vi "ReadConcTempPressureVer08.vi"() -> ()   [LabVIEW 2011]
uses:
  <vilib>/Utility/error.llb/DialogType.ctl
  <vilib>/Analysis/NI_AALBase.lvlib
panel:
  out "CavityTemperature":dbl
  out "CavityPressure":dbl
  in  "Measurment Type":T1(ring)=enum."Particles Measurement"
  out "CPCconc":dbl=nan
  out "Smps Setting String":string
  out "Saving in Progress":i32(slide) caption="Saving" scale=0.0..9.0
  out "P (Hectopascal)":dbl=1014.187137206139 format="%#.2f"
  out "Mean P":dbl=1014.4104948184322 format="%.1f"
  out "Std Error P (%)":dbl=0.009142669652284326 format="%.2f"
  out "Number Samples of Press.":dbl format="%.1f"
  out "Std error Press. to file (hpas)":dbl format="%.2f"
  out "Mean Press. to file (hpas)":dbl format="%.2f"
  in  "Std Press. error tolerance(%)":dbl=0.1 format="%.1f"
  out "Pressure Graph":waveform(dbl)[](graph)=[{"t0"=timestamp(3472445026.4531226 s since 1904-01-01), "dt"=1.0, "Y"=[1014.187137206139]}, {"t0"=timestamp(3472445026.4531226 s since 1904-01-01), "dt"=1.0, "Y"=[1014.4104948184322]}] caption="Waveform Chart"
  out "Temp (C)":dbl=23.130823558220463 format="%#.2f"
  out "Mean Temp":dbl=23.127451250466187 format="%.2f"
  out "Std Error T (%)":dbl=0.012599717898815081 format="%.2f"
  out "Number Samples of Temp":dbl format="%.1f"
  out "Std error Temp to file (deg)":dbl format="%.1f"
  out "Mean Temp to file (deg)":dbl format="%#.0f"
  in  "Std Temp error tolerance(%)":dbl=0.1 format="%.1f"
  out "Temperature Graph":waveform(dbl)[](graph)=[{"t0"=timestamp(3472445026.4531226 s since 1904-01-01), "dt"=1.0, "Y"=[23.130823558220463]}, {"t0"=timestamp(3472445026.4531226 s since 1904-01-01), "dt"=1.0, "Y"=[23.127451250466187]}] caption="Waveform Chart"
  in  "CPC port":refnum<visa-resource-name>="COM1"
  out "Conc. (N/cm^3)":dbl=nan format="%.1f"
  out "Mean Conc.":dbl=nan format="%.1f"
  out "Std Error Conc. (%)":dbl=nan format="%.2f"
  out "Number Samples of Conc.":dbl format="%.1f"
  out "Std error to file (N/cm^3)":dbl format="%.1f"
  out "Mean conc. to file (N/cm^3)":dbl format="%.2f"
  out "output array 2":dbl[](array[numeric])
  out "output 2":dbl
  out "output 1":dbl
  out "Std Error Concentration":dbl=nan format="%.1f"
  in  "Std Conc. error tolerance(%)":dbl=1.0 format="%.1f"
  out "Std Concentration":dbl=nan format="%.1f"
  out "output array":dbl[](array[numeric])=[nan, nan, nan, nan, nan, nan, nan, nan, nan, nan, nan, 0.0, 0.0, 0.0, 0.0, 1.0, 1.0, 1.0, 0.0, 0.0, 0.0, 0.0, 0.0, 0.0, 0.0, 0.0, 0.0, nan, nan, nan]
  in  "Running Average Time(sec)":i32=30
  out "Particle Concentration from CPC":waveform(dbl)[](graph)=[{"t0"=timestamp(3472445026.4531226 s since 1904-01-01), "dt"=1.0, "Y"=[nan]}, {"t0"=timestamp(3472445026.4531226 s since 1904-01-01), "dt"=1.0, "Y"=[nan]}] caption="Waveform Chart"
  in  "OK":bool
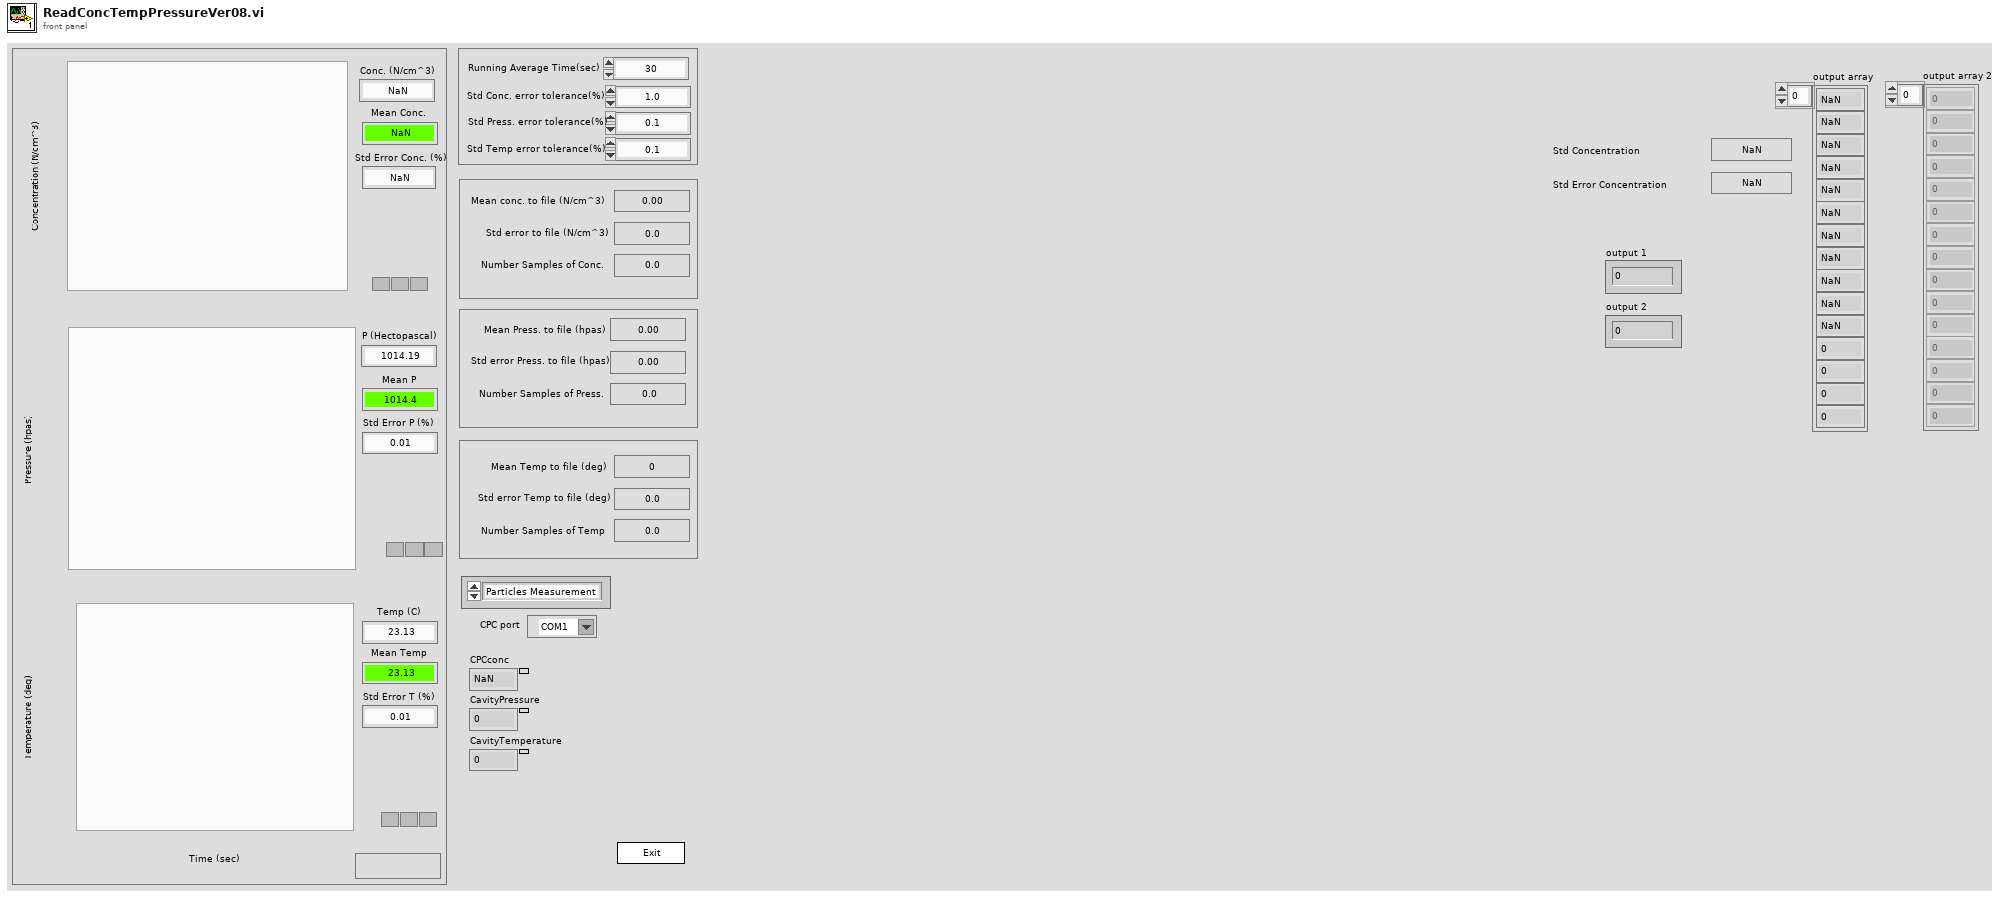
[diagram p1: front panel]
types:
  T1 = enum16{"Gas Measurement", "Particles Measurement", "SMPS scan"}
  T2 = enum32{"invalid app kind", "Development System", "Run Time System", "Student Edition", "Embedded LabVIEW", "Evaluation", "Custom"}
  T3 = enum32{"Invalid", "Standard", "Closed", "Hidden", "Minimized", "Maximized"}
  T4 = cluster{"Core":cluster{"Current VI Reference":refnum<vi>, "Close Panel on Exit?":bool}, dbl[], "Running Average Time(sec)":i32, dbl[], "element":dbl, "dimension size":i32, "input file":path, "input file":path, "dup CPC port":refnum<visa-resource-name>, "CPC model":string, "input file":path, "input file":path, cluster{dbl[], dbl[], "element":dbl}, cluster{dbl[], dbl[], "element":dbl}}
  T5 = typedef "DialogType.ctl" = u16
  T6 = cluster{"Current VI Reference":refnum<vi>, "Close Panel on Exit?":bool}
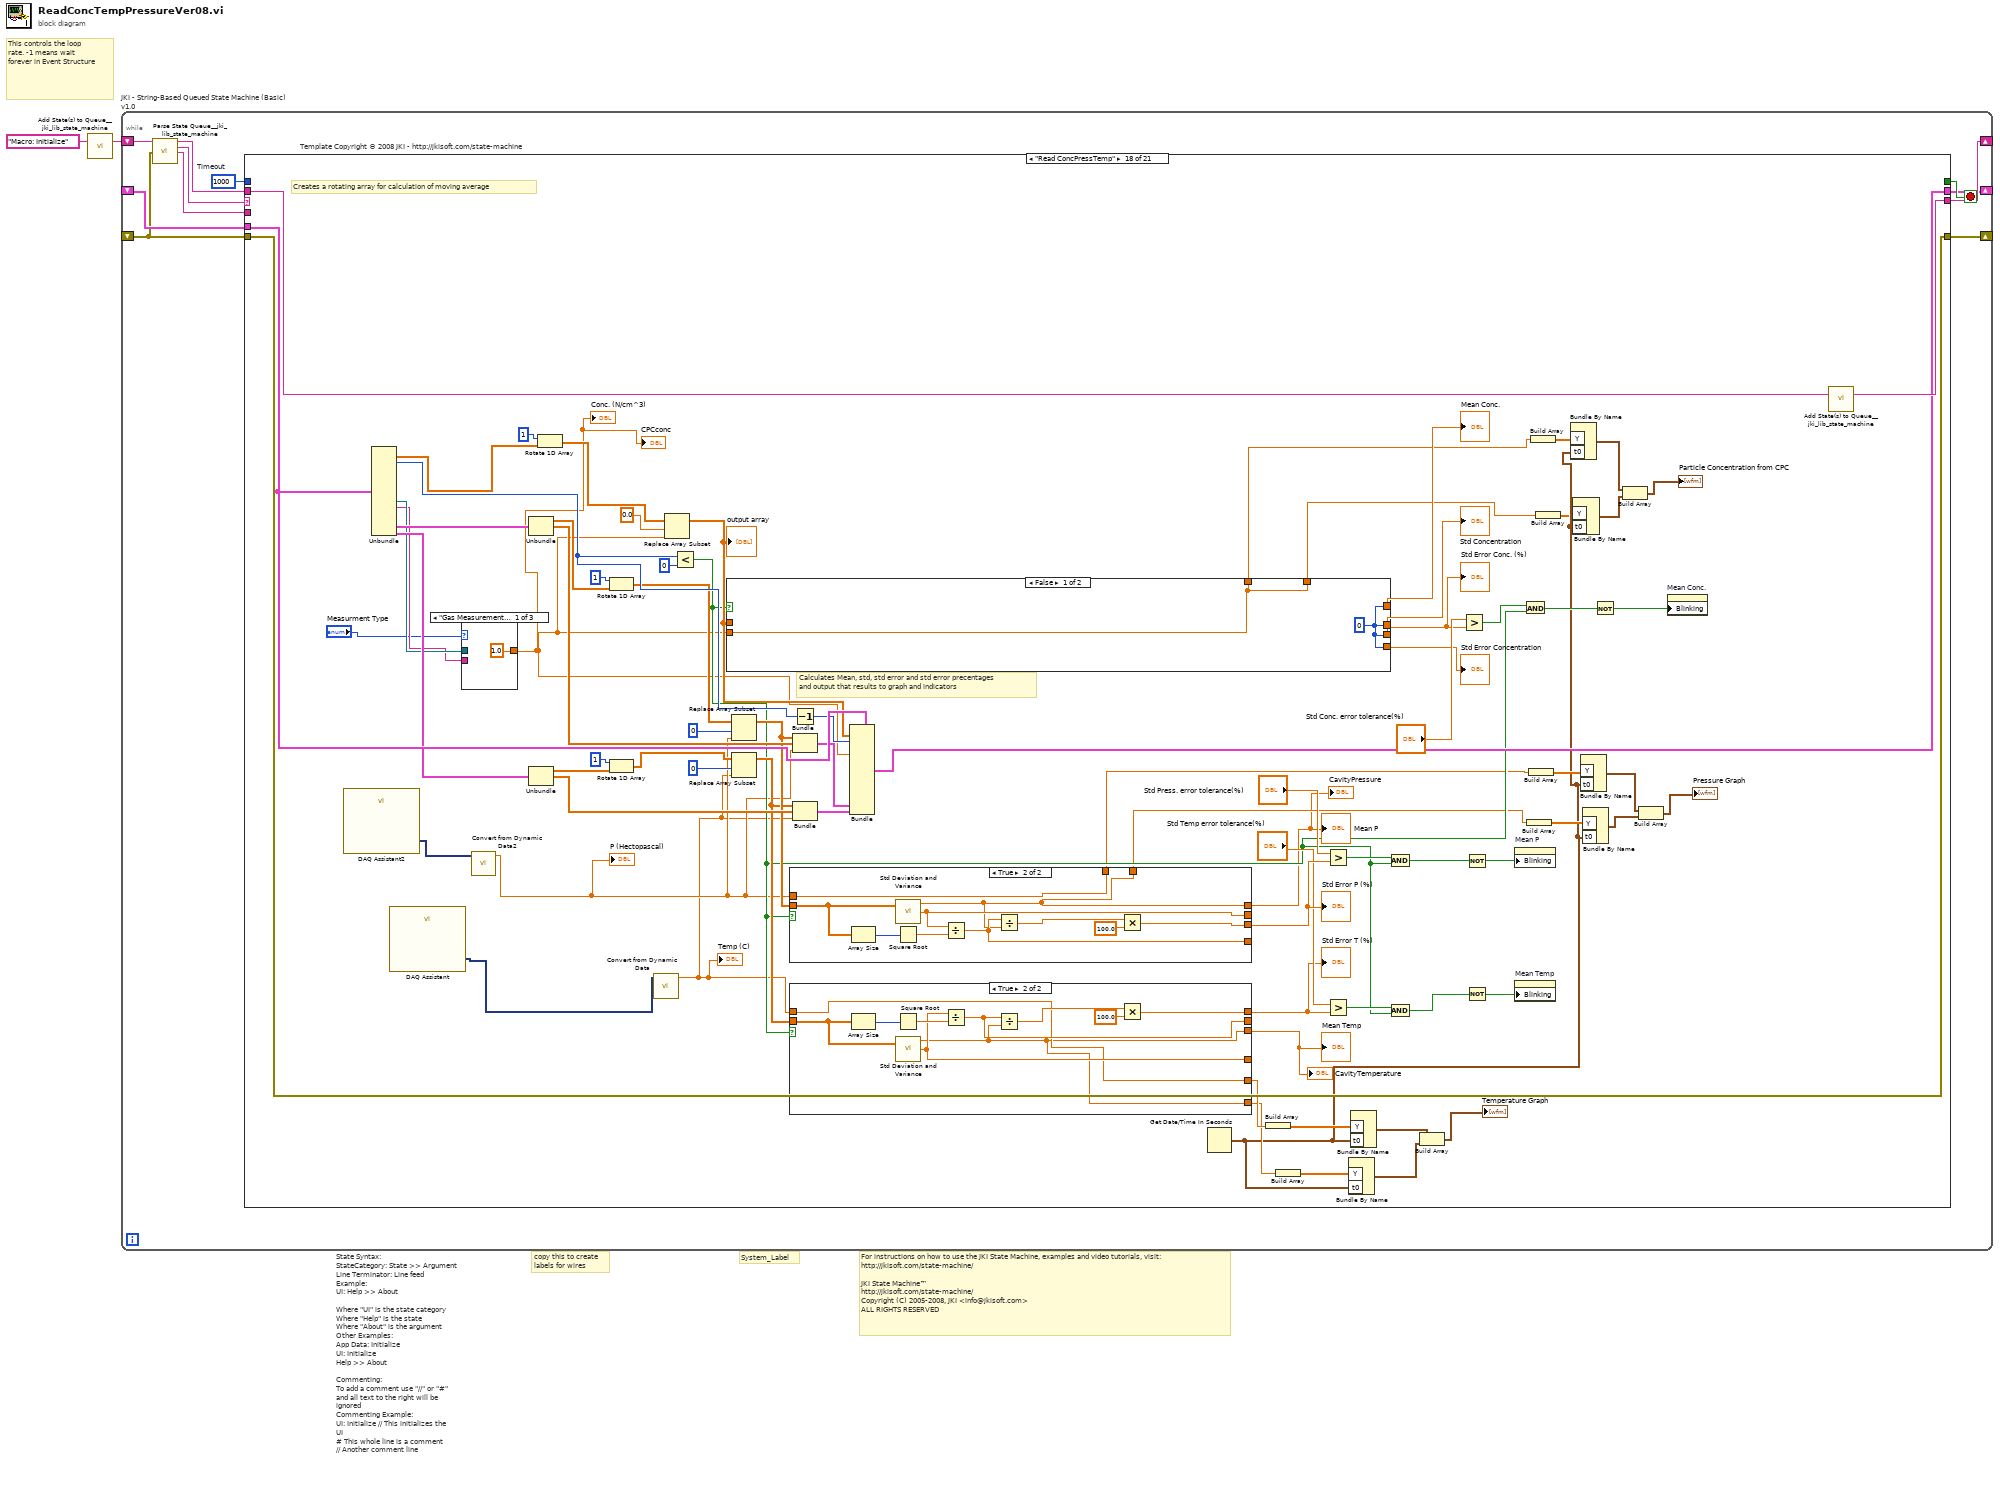
[diagram p0: block diagram]
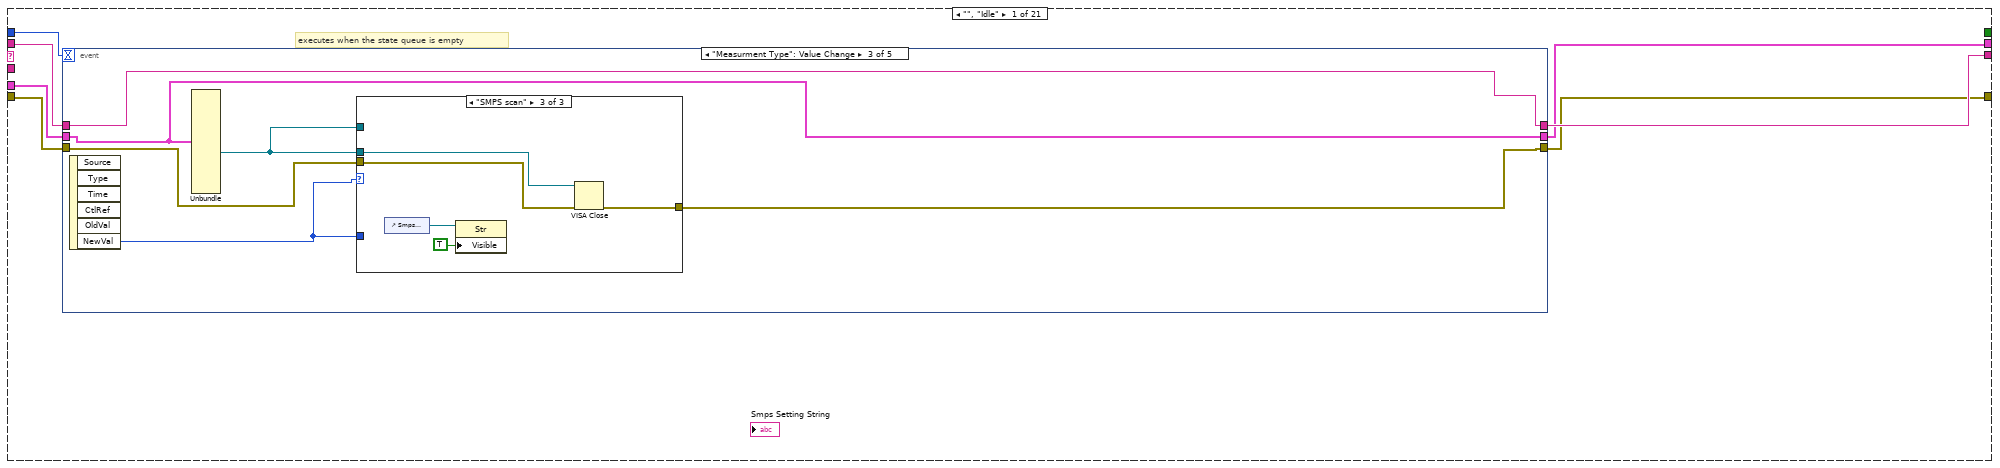
[diagram p2: hidden frame]
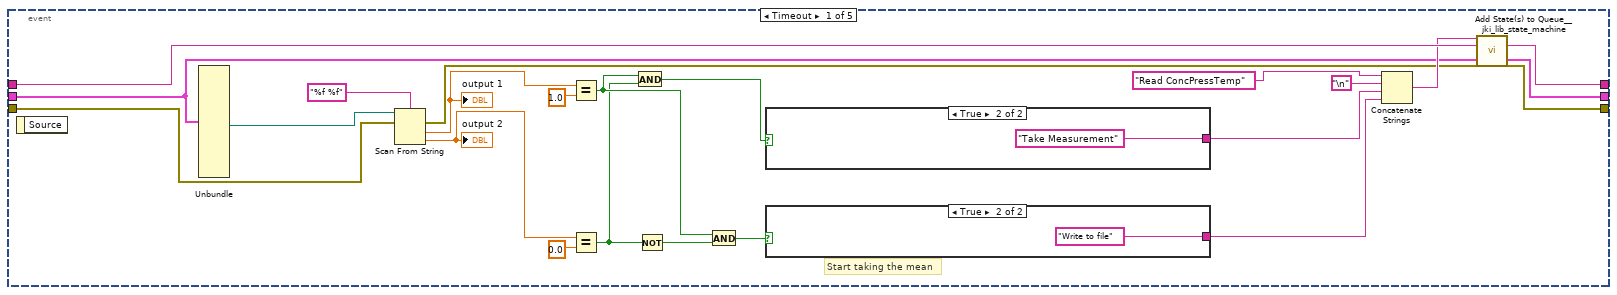
[diagram p3: hidden frame]
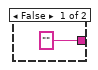
[diagram p4: hidden frame]
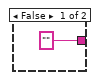
[diagram p5: hidden frame]
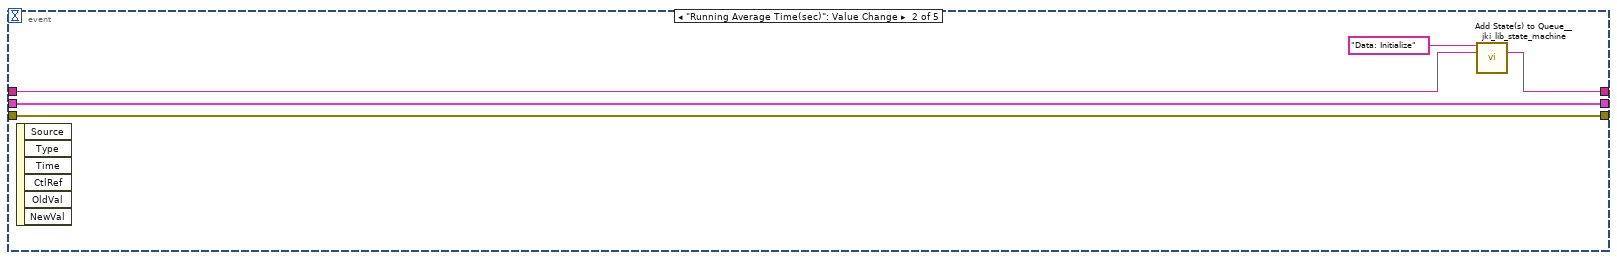
[diagram p6: hidden frame]
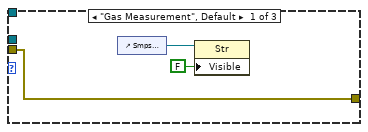
[diagram p7: hidden frame]
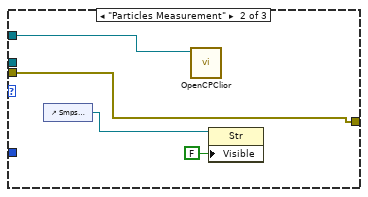
[diagram p8: hidden frame]
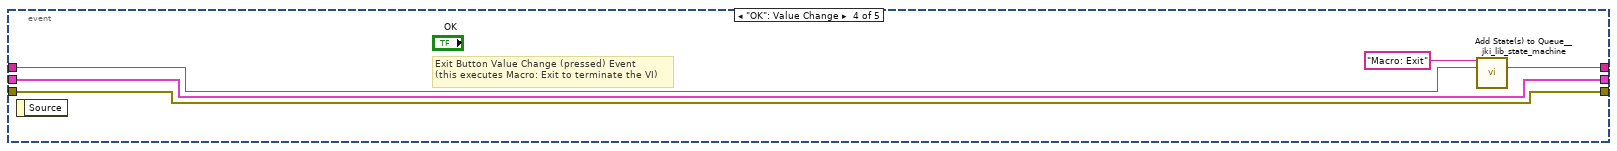
[diagram p9: hidden frame]
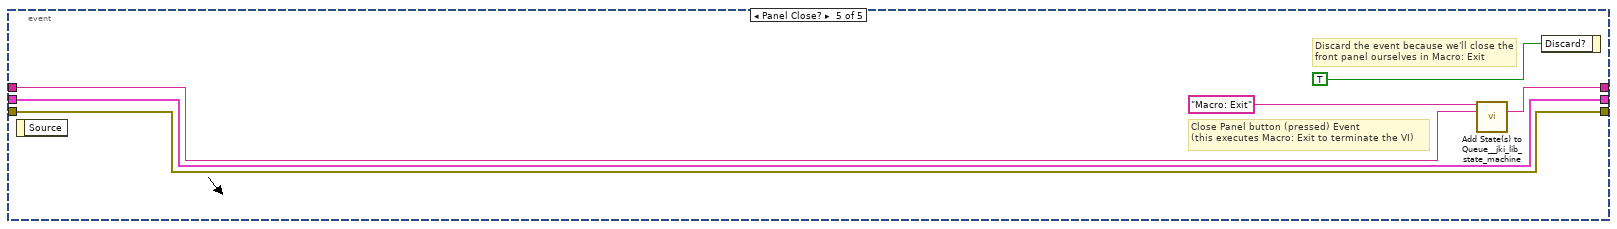
[diagram p10: hidden frame]
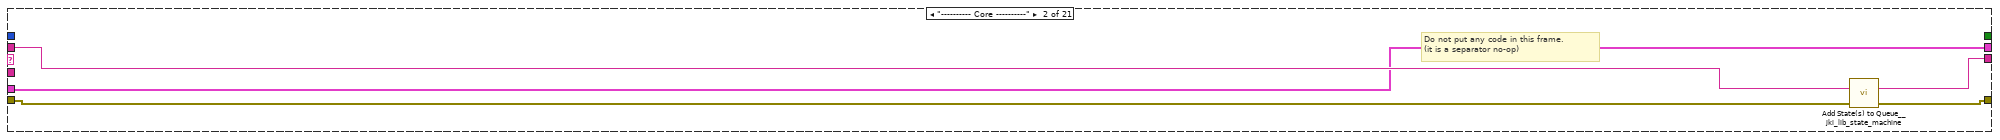
[diagram p11: hidden frame]
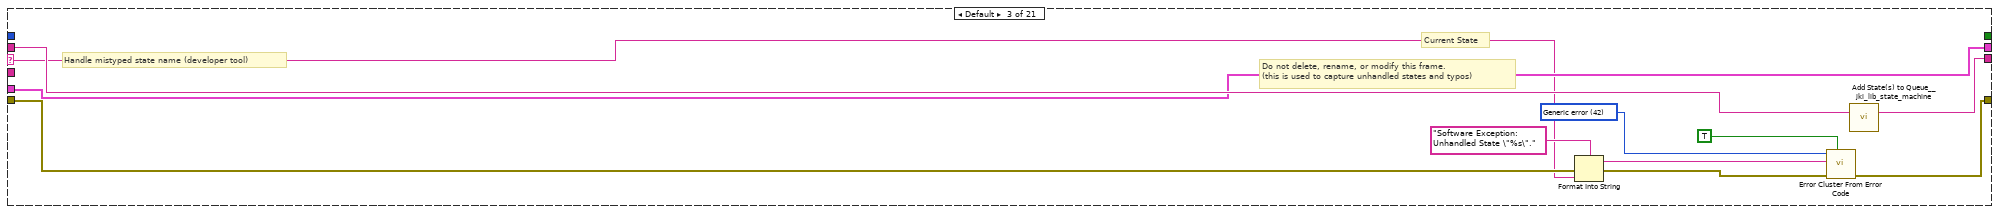
[diagram p12: hidden frame]
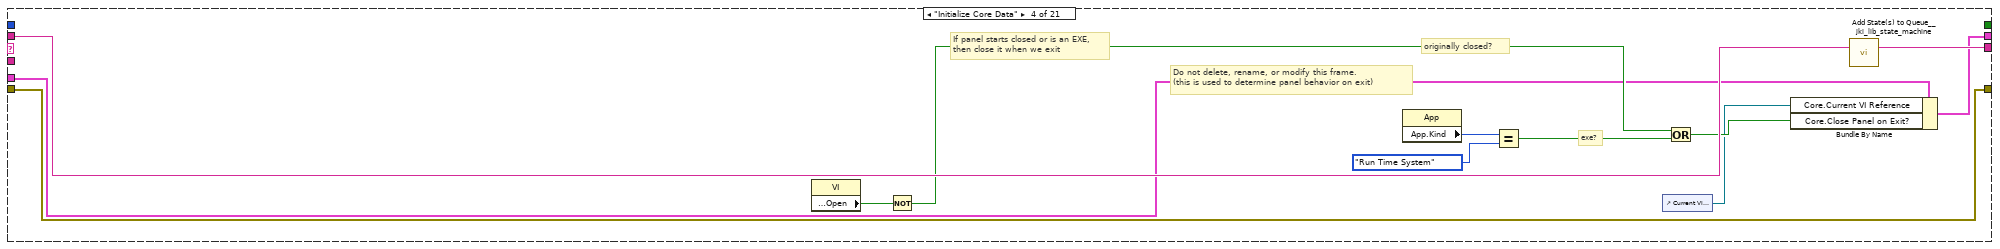
[diagram p13: hidden frame]
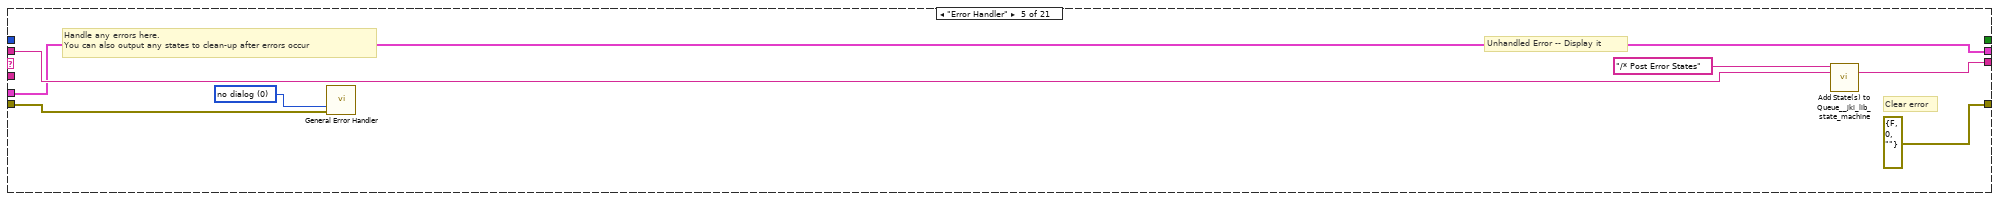
[diagram p14: hidden frame]
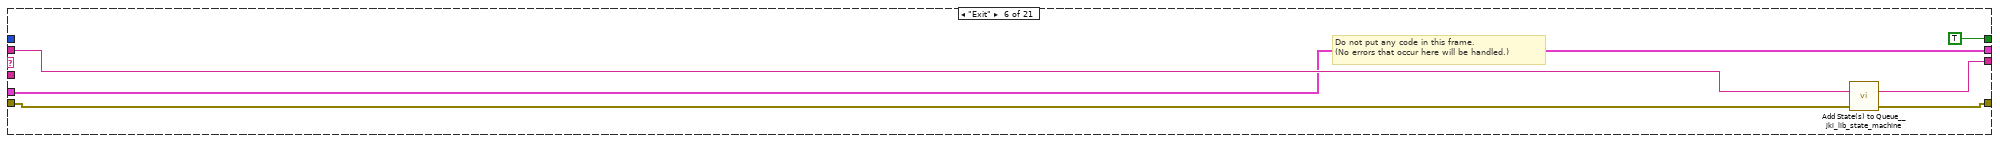
[diagram p15: hidden frame]
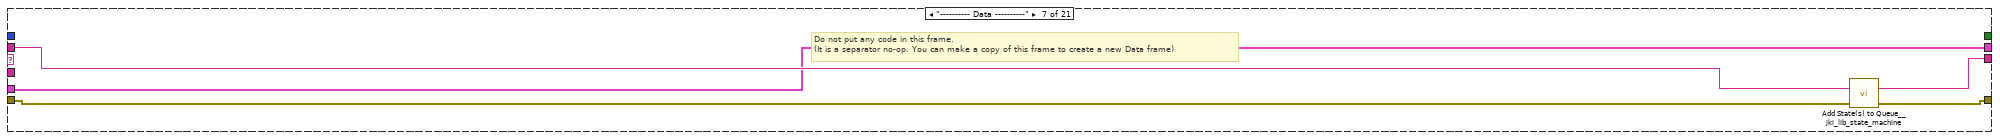
[diagram p16: hidden frame]
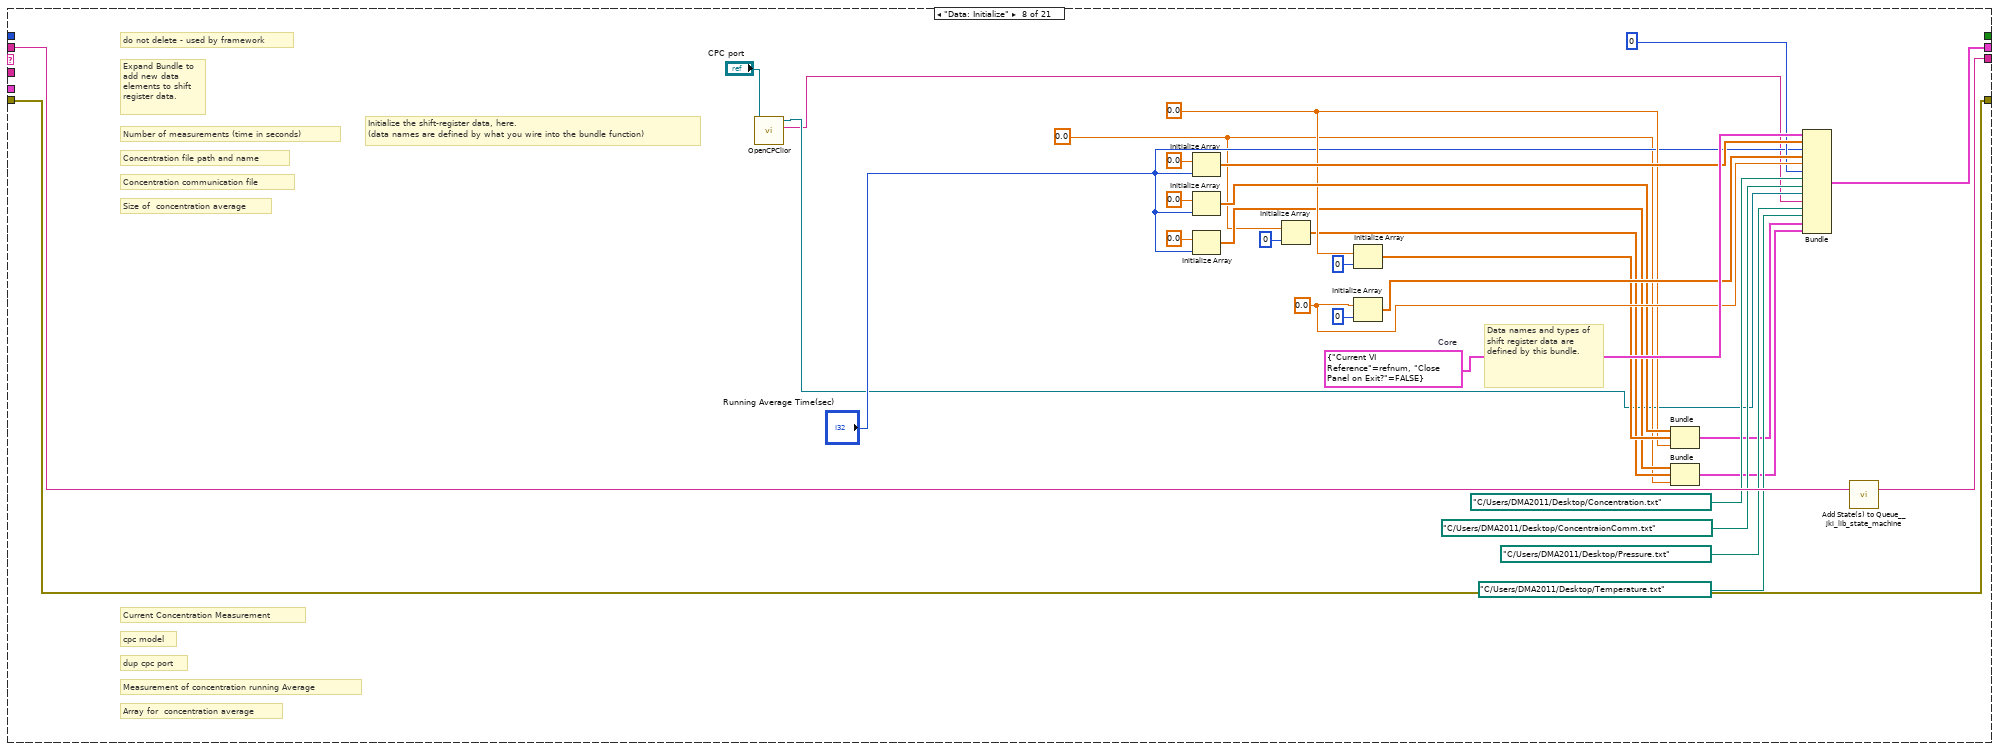
[diagram p17: hidden frame]
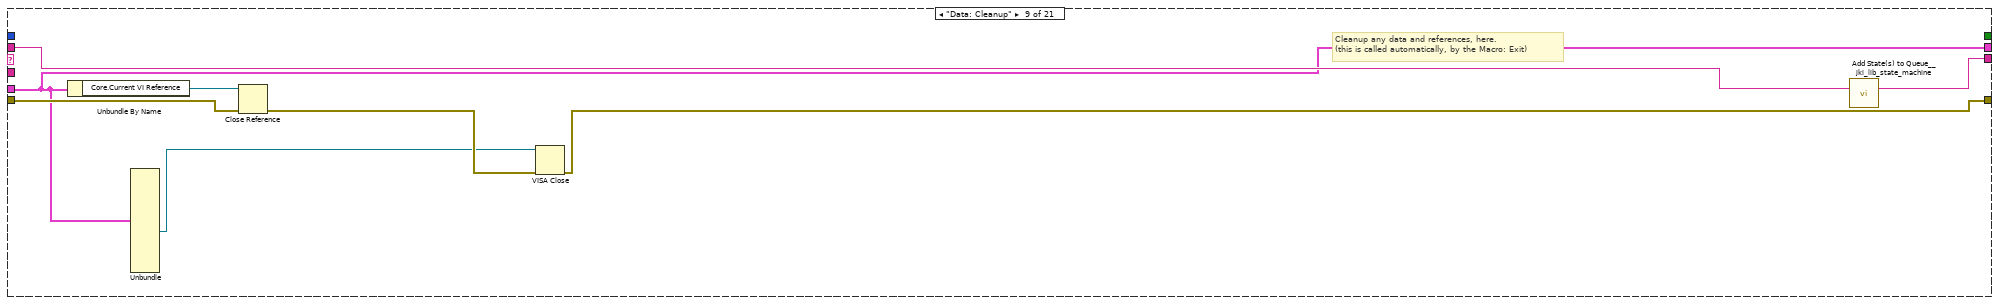
[diagram p18: hidden frame]
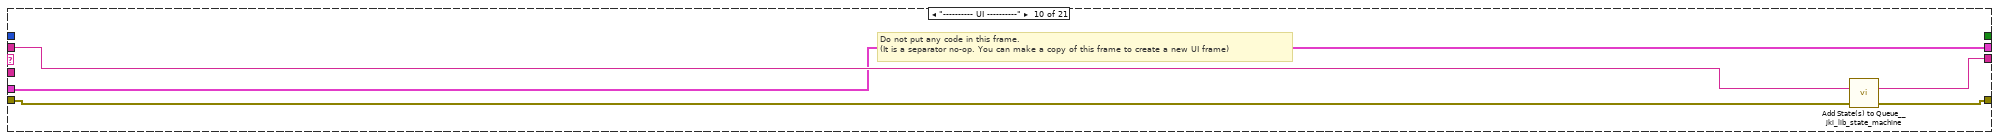
[diagram p19: hidden frame]
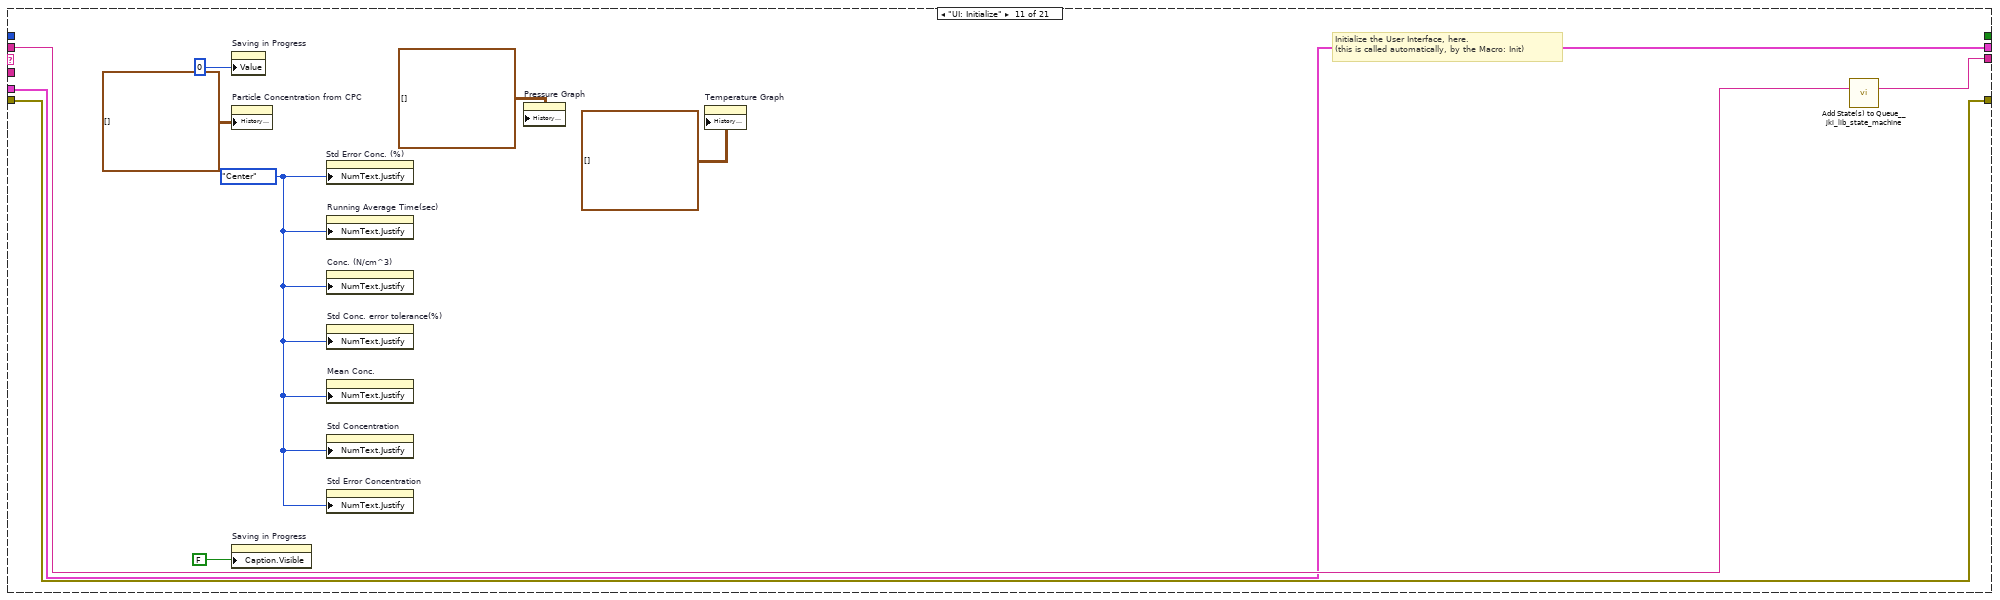
[diagram p20: hidden frame]
diagram:
  # "For instructions on how to use the JKI State Machine, examples and video tutorials, visit:\nhttp://jkisoft.com/state-machine/\n\nJKI State Machine™\nhttp://jkisoft.com/state-machine/\nCopyright (C) 2005-2008, JKI <info@jkisoft.com>\nALL RIGHTS RESERVED"
  # "State Syntax:\nStateCategory: State >> Argument\nLine Terminator: Line feed\nExample:\nUI: Help >> About\n\nWhere \"UI\" is the state category\nWhere \"Help\" is the state\nWhere \"About\" is the argument\nOther Examples:\nApp Data: Initialize\nUI: Initialize\nHelp >> About\n\nCommenting:\nTo add a comment use \"//\" or \"#\" and all text to the right will be ignored\nCommenting Example:\nUI: Initialize // This initializes the UI\n# This whole line is a comment\n// Another comment line"
  # "copy this to create labels for wires"
  # "This controls the loop rate. -1 means wait forever in Event Structure"
  # "System_Label"
  n1 = call <vilib>:"Add State(s) to Queue__jki_lib_state_machine.vi"("State(s) in (\"\")"="Macro: Initialize") -> ("States Out"=w2:string)  [unwired: 14 in]
  n2 = while "JKI - String-Based Queued State Machine (Basic) v1.0" {
    shift-right: [w6] -> _
    shift-left: _ -> [w5]
    shift-right: [w9] -> _
    shift-left: _ -> [w3]
    shift-right: [w8] -> _
    shift-left: w2 -> [w10]
    stop <- w7 stop-if-true
    w4 = 1000  # Timeout
    # "Template Copyright © 2008 JKI - http://jkisoft.com/state-machine"
    n3 = call <vilib>:"Parse State Queue__jki_lib_state_machine.vi"("State Queue"=w10, "Error In (no error)"=w3) -> ("Remaining States"=w12:string, "Current State"=w13:string, "Arguments"=w11:string)  [unwired: 11 in]
    n4 = case shown="\"Read ConcPressTemp\"" w13 {
      selector: w13 -> [_ _ w84 _ _ _ _ _ _ _ _ _ _ _ _ _ _ _ _ _ _]
      tunnel: w12 -> [w20 w83 w88 w106 w113 w118 w122 w153 w161 w165 w175 w181 w192 w218 w223 w233 w237 w317 w362 w392 w452]
      tunnel: w11 -> [_ _ _ _ _ _ _ _ _ _ _ w176 w186 _ _ _ _ _ _ _ _]
      tunnel: w5 -> [w18 w80 w86 w97 w110 w116 w119 _ w155 w162 w173 w179 w188 w215 w220 w230 w234 w313 w359 w386 w441]
      tunnel: [w17 w81 w90 w103 errorcluster {"status"=FALSE, "code"=0, "source"=""} ("error out") w115 w120 w150 w156 w163 w172 w177 w189 w216 w221 w231 w235 w315 w360 w390 w415] -> w9
      tunnel: w3 -> [w16 w81 w89 w103 w109 w115 w120 w150 w158 w163 w172 w178 w190 w216 w221 w231 w235 w315 w360 w390 w430]
      tunnel: [w19 w82 w87 w105 w112 w117 w121 w152 w160 w164 w174 w180 w191 w217 w222 w232 w236 w316 w361 w391 w451] -> w8
      tunnel: [_ _ _ _ _ TRUE _ _ _ _ _ _ _ _ _ _ _ _ _ _ _] -> w7
      tunnel: [w15 w80 w86 w104 w110 w116 w119 w151 w155 w162 w173 w179 w188 w215 w220 w230 w234 w314 w359 w385 w440] -> w6
      tunnel: w4 -> [w14 _ _ _ _ _ _ _ _ _ _ _ _ _ _ _ _ _ _ _ _]
      frame "", "Idle" {
        # "executes when the state queue is empty"
        n5 = event shown="[2] \"Measurment Type\": Value Change" {
          selector: _ -> [_ _ _ _ _]
          dyn-events: _ -> [_ _ _ _ _]
          timeout: w14 -> [_ _ _ _ _]
          tunnel: w20 -> [w41 w50 w53 w73 w79]
          tunnel: [w40 w49 w53 w72 w78] -> w19
          tunnel: w18 -> [w24 w47 w52 w70 w76]
          tunnel: [w21 w48 w55 w71 w77] -> w17
          tunnel: w16 -> [w22 w48 w56 w71 w77]
          tunnel: [w24 w47 w52 w70 w76] -> w15
          event Timeout {
            # "Start taking the mean"
            n6 = event-data() -> ()  [unwired: 1 in, 1 out]
            n7 = Unbundle(w24) -> ("input file"=w23:path)  [unwired: 13 out]
            n8 = Scan From String("%f %f" ("format string"), w23, w22) -> (w21:errorcluster, output 1=w38:dbl, output 2=w35:dbl)  [unwired: 2 in, 1 out]
            "output 1" <- w38
            "output 2" <- w35
            n9 = Equal?(x=w38, y=1.0) -> (x = y?=w29:bool)
            n10 = Equal?(x=w35, y=0.0) -> (x = y?=w27:bool)
            n11 = And(x=w29, y=w27) -> (x .and. y?=w34:bool)
            n12 = Not(x=w27) -> (.not. x?=w28:bool)
            n13 = And(x=w29, y=w28) -> (x .and. y?=w26:bool)
            n14 = case shown="True" w34 {
              tunnel: ["" ("State(s) in Front (\"\")") "Take Measurement" ("State(s) in Front (\"\")")] -> w30
              frame False {
              }
              frame True {
              }
            }
            n15 = case shown="True" w26 {
              tunnel: ["" ("State(s) in Front (\"\")") "Write to file" ("State(s) in Front (\"\")")] -> w25
              frame False {
              }
              frame True {
              }
            }
            n16 = Concatenate Strings("Read ConcPressTemp" ("State(s) in Front (\"\")"), "\n", w30, w25) -> (w33:string)
            n17 = call <vilib>:"Add State(s) to Queue__jki_lib_state_machine.vi"("State(s) in Front (\"\")"=w33, "State(s) in (\"\")"=w41) -> ("States Out"=w40:string)  [unwired: 13 in]
          }
          event "Running Average Time(sec)": Value Change {
            n18 = event-data() -> ()  [unwired: 1 in, 6 out]
            n19 = call <vilib>:"Add State(s) to Queue__jki_lib_state_machine.vi"("State(s) in Front (\"\")"="Data: Initialize" ("State(s) in Front (\"\")"), "State(s) in (\"\")"=w50) -> ("States Out"=w49:string)  [unwired: 13 in]
          }
          event "Measurment Type": Value Change {
            n20 = event-data() -> ("NewVal"=w51:T1)  [unwired: 1 in, 5 out]
            n21 = Unbundle(w52) -> ("dup CPC port"=w54:refnum<visa-resource-name>)  [unwired: 13 out]
            n22 = case shown="\"SMPS scan\"" w51 {
              tunnel: w54 -> [_ _ w68]
              tunnel: w56 -> [w59 w62 w67]
              tunnel: [w59 w62 w66] -> w55
              tunnel: w54 -> [_ w63 _]
              tunnel: w51 -> [_ _ _]
              frame "Gas Measurement", Default {
                n23 = control-ref of="Smps Setting String"() -> (w57:refnum<vi>)
                n24 = property on="Property Node" class="Str"(reference=w57, "Visible"=FALSE) -> ()  [unwired: 1 in, 2 out]
              }
              frame "Particles Measurement" {
                n25 = control-ref of="Smps Setting String"() -> (w61:refnum<vi>)
                n26 = call "OpenCPClior.vi"("CPC port"=w63) -> ()  [unwired: 8 in, 3 out]
                n27 = property on="Property Node" class="Str"(reference=w61, "Visible"=FALSE) -> ()  [unwired: 1 in, 2 out]
              }
              frame "SMPS scan" {
                n28 = control-ref of="Smps Setting String"() -> (w65:refnum<vi>)
                n29 = property on="Property Node" class="Str"(reference=w65, "Visible"=TRUE) -> ()  [unwired: 1 in, 2 out]
                n30 = VISA Close(VISA resource name=w68, error in (no error)=w67) -> (error out=w66:errorcluster)
              }
            }
          }
          event "OK": Value Change {
            # "Exit Button Value Change (pressed) Event\n(this executes Macro: Exit to terminate the VI)"
            n31 = event-data() -> ()  [unwired: 1 in, 1 out]
            n32 = call <vilib>:"Add State(s) to Queue__jki_lib_state_machine.vi"("State(s) in Front (\"\")"="Macro: Exit", "State(s) in (\"\")"=w73) -> ("States Out"=w72:string)  [unwired: 13 in]
          }
          event Panel Close? {
            # "Discard the event because we'll close the front panel ourselves in Macro: Exit"
            # "Close Panel button (pressed) Event\n(this executes Macro: Exit to terminate the VI)"
            n33 = event-data() -> ()  [unwired: 1 in, 1 out]
            n34 = call <vilib>:"Add State(s) to Queue__jki_lib_state_machine.vi"("State(s) in Front (\"\")"="Macro: Exit", "State(s) in (\"\")"=w79) -> ("States Out"=w78:string)  [unwired: 13 in]
            n35 = event-data("Discard?"=TRUE) -> ()  [unwired: 1 in, 1 out]
          }
        }
      }
      frame "---------- Core ----------" {
        # "Do not put any code in this frame.\n(it is a separator no-op)"
        n36 = call <vilib>:"Add State(s) to Queue__jki_lib_state_machine.vi"("State(s) in (\"\")"=w83) -> ("States Out"=w82:string)  [unwired: 14 in]
      }
      frame Default {
        w93 = 42 items=["No error", "Argument error", "Memory is full", "Out of zone", "End of file", "File already open", "Generic file I/O error", "File not found", "File permission error", "Disk is full", "Duplicate path", "Too many files open", "System feature not enabled", "Resource file not found", "Cannot add resource", "Resource not found", "Image not found", "Image memory error", "Pen does not exist", "Config type invalid", "Config token not found", "Config parse error", "Config memory error", "Bad external code format", "Bad external code offset", "External code not present", "Null window", "Destroy window error", "Null menu", "Print aborted", "Bad print record", "Print driver error", "Windows error during printing", "Memory error during printing", "Print dialog error", "Generic print error", "Invalid device refnum", "Device not found", "Device parameter error", "Device unit error", "Cannot open device", "Device call aborted", "Generic error", "Cancelled by user", "Object ID too low", "Object ID too high", "Object not in heap", "Unknown heap", "Unknown object (invalid DefProc)", "Unknown object (DefProc not in table)", "Message out of range", "Invalid (null) method", "Unknown message", "Manager call not supported", "Bad address", "Network operation in progress", "Network operation timed out", "Connection is busy", "Network attribute not supported", "Network error", "Address in use", "System out of memory", "Connection aborted", "Connection refused", "Not connected", "Already connected", "Connection closed", "Initialization error (interapplication manager)", "Bad occurrence", "Wait on unbound occurrence handler", "Occurrence queue overflow", "Datalog type conflict", "Unused", "Unrecognized type (interapplication manager)", "Memory corrupt", "Failed to make temporary DLL", "Old CIN version", "Drag socket not found", "Failed to load drop-object", "Failed to register OLE object", "Failed to release OLE object", "Format specifier type mismatch", "Unknown format specifier", "Too few format specifiers", "Too many format specifiers", "Scan failed", "Newer CIN version", "Error converting to variant", "Runtime menu error", "Password tampered", "Variant attribute not found", "Incompatible variant data type", "Event data is not available", "Event Store is not present", "Occurrence is not found", "Event Queue is not created", "Event info is not available", "Refnum passed is NULL", "Error retrieving Class GUID", "Error retrieving CoClass GUID", "Error retrieving TypeLib GUID.", "Bad built application magic bytes.", "Specific driver is different from the specific driver associated with the Logical Name.", "There is no session opened to the class driver.", "Max Error", "MAX - Error with config objects", "MAX - Error loading configuration", "MAX - Group not supported"]
        # "Current State"
        # "Do not delete, rename, or modify this frame.\n(this is used to capture unhandled states and typos)"
        # "Handle mistyped state name (developer tool)"
        n37 = Format Into String(format string="Software Exception: Unhandled State \"%s\"." ("message"), error in=w89, w84) -> (resulting string=w92:string, error out=w91:errorcluster)  [unwired: 1 in]
        n38 = call <vilib>:"Error Cluster From Error Code.vi"("show call chain? (False)"=TRUE, "error in (no error)"=w91, "error message (\"\")"=w92, "error code (0)"=w93) -> ("error out"=w90:errorcluster)  [unwired: 5 in]
        n39 = call <vilib>:"Add State(s) to Queue__jki_lib_state_machine.vi"("State(s) in (\"\")"=w88) -> ("States Out"=w87:string)  [unwired: 14 in]
      }
      frame "Initialize Core Data" {
        # "Do not delete, rename, or modify this frame.\n(this is used to determine panel behavior on exit)"
        # "originally closed?"
        # "exe?"
        # "If panel starts closed or is an EXE, then close it when we exit"
        n40 = property class="VI"() -> ("Front Panel.Open"=w102:bool)  [unwired: 2 in, 2 out]
        n41 = Not(x=w102) -> (.not. x?=w99:bool)
        n42 = property class="App"() -> ("App.Kind"=w101:T2)  [unwired: 2 in, 2 out]
        n43 = Equal?(x=w101, y=T2."Run Time System" ("Application:Kind")) -> (x = y?=w98:bool)
        n44 = control-ref of="Current VI Reference"() -> (w95:refnum<vi>)
        n45 = Or(x=w99, y=w98) -> (x .or. y?=w96:bool)
        n46 = Bundle By Name(cluster=w97, "Core.Current VI Reference"=w95, "Core.Close Panel on Exit?"=w96) -> (w104:T4)
        n47 = call <vilib>:"Add State(s) to Queue__jki_lib_state_machine.vi"("State(s) in (\"\")"=w106) -> ("States Out"=w105:string)  [unwired: 14 in]
      }
      frame "Error Handler" {
        w107 = T5 0 items=["no dialog", "OK message", "continue or stop message", "OK message + warnings", "continue/stop + warnings"] ("type of dialog (OK msg:1)")
        # "Unhandled Error -- Display it"
        # "Handle any errors here.\nYou can also output any states to clean-up after errors occur"
        # "Clear error"
        n48 = call <vilib>:"General Error Handler.vi"("type of dialog (OK msg:1)"=w107, "error in (no error)"=w109) -> ()  [unwired: 9 in, 5 out]
        n49 = call <vilib>:"Add State(s) to Queue__jki_lib_state_machine.vi"("State(s) in Front (\"\")"="/* Post Error States", "State(s) in (\"\")"=w113) -> ("States Out"=w112:string)  [unwired: 13 in]
      }
      frame "Exit" {
        # "Do not put any code in this frame.\n(No errors that occur here will be handled.)"
        n50 = call <vilib>:"Add State(s) to Queue__jki_lib_state_machine.vi"("State(s) in (\"\")"=w118) -> ("States Out"=w117:string)  [unwired: 14 in]
      }
      frame "---------- Data ----------" {
        # "Do not put any code in this frame.\n(It is a separator no-op. You can make a copy of this frame to create a new Data frame)"
        n51 = call <vilib>:"Add State(s) to Queue__jki_lib_state_machine.vi"("State(s) in (\"\")"=w122) -> ("States Out"=w121:string)  [unwired: 14 in]
      }
      frame "Data: Initialize" {
        w126 = 0.0 ("element")
        w133 = 0.0 ("element")
        w144 = 0.0 ("element")
        w149 = T6 {"Current VI Reference"=refnum, "Close Panel on Exit?"=FALSE}  # Core
        # "cpc model"
        # "dup cpc port"
        # "Concentration communication file"
        # "Concentration file path and name"
        # "Number of measurements (time in seconds)"
        # "Current Concentration Measurement"
        # "Size of  concentration average"
        # "Array for  concentration average"
        # "Measurement of concentration running Average"
        # "do not delete - used by framework"
        # "Expand Bundle to add new data elements to shift register data."
        # "Data names and types of shift register data are defined by this bundle."
        # "Initialize the shift-register data, here.\n(data names are defined by what you wire into the bundle function)"
        n52 = call "OpenCPClior.vi"("CPC port"="CPC port") -> ("CPC model"=w123:string, "dup CPC port"=w124:refnum<visa-resource-name>)  [unwired: 8 in, 1 out]
        n53 = Initialize Array(0.0 ("element"), "Running Average Time(sec)") -> (w147:dbl[])
        n54 = Initialize Array(0.0 ("element"), "Running Average Time(sec)") -> (w137:dbl[])
        n55 = Initialize Array(0.0 ("element"), "Running Average Time(sec)") -> (w130:dbl[])
        n56 = Initialize Array(w126, 0 ("dimension size")) -> (w127:dbl[])
        n57 = Initialize Array(w133, 0 ("dimension size")) -> (w134:dbl[])
        n58 = Initialize Array(w144, 0 ("dimension size")) -> (w145:dbl[])
        n59 = Bundle(w137, w134, "element"=w133) -> (w136:cluster{dbl[], dbl[], "element":dbl})  [unwired: 1 in]
        n60 = Bundle(w130, w127, "element"=w126) -> (w132:cluster{dbl[], dbl[], "element":dbl})  [unwired: 1 in]
        n61 = Bundle("Core"=w149, w147, "Running Average Time(sec)"="Running Average Time(sec)", w145, "element"=w144, "dimension size"=0, "input file"=path "C:/Users/DMA2011/Desktop/Concentration.txt", "input file"=path "C:/Users/DMA2011/Desktop/ConcentraionComm.txt", "dup CPC port"=w124, "CPC model"=w123, "input file"=path "C:/Users/DMA2011/Desktop/Pressure.txt", "input file"=path "C:/Users/DMA2011/Desktop/Temperature.txt", w136, w132) -> (w151:T4)  [unwired: 1 in]
        n62 = call <vilib>:"Add State(s) to Queue__jki_lib_state_machine.vi"("State(s) in (\"\")"=w153) -> ("States Out"=w152:string)  [unwired: 14 in]
      }
      frame "Data: Cleanup" {
        # "Cleanup any data and references, here.\n(this is called automatically, by the Macro: Exit)"
        n63 = Unbundle By Name(w155) -> ("Core.Current VI Reference"=w159:refnum<vi>)
        n64 = Unbundle(w155) -> ("dup CPC port"=w154:refnum<visa-resource-name>)  [unwired: 13 out]
        n65 = Close Reference(reference=w159, error in (no error)=w158) -> (error out=w157:errorcluster)
        n66 = VISA Close(VISA resource name=w154, error in (no error)=w157) -> (error out=w156:errorcluster)
        n67 = call <vilib>:"Add State(s) to Queue__jki_lib_state_machine.vi"("State(s) in (\"\")"=w161) -> ("States Out"=w160:string)  [unwired: 14 in]
      }
      frame "---------- UI ----------" {
        # "Do not put any code in this frame.\n(It is a separator no-op. You can make a copy of this frame to create a new UI frame)"
        n68 = call <vilib>:"Add State(s) to Queue__jki_lib_state_machine.vi"("State(s) in (\"\")"=w165) -> ("States Out"=w164:string)  [unwired: 14 in]
      }
      frame "UI: Initialize" {
        w169 = enum16{"Left", "Center", "Right"}."Center" ("Numeric Text.Justification")
        # "Initialize the User Interface, here.\n(this is called automatically, by the Macro: Init)"
        n69 = property on="Saving in Progress" class="Slide (strict)"("Value"=0 ("Saving in Progress")) -> ()  [unwired: 2 in, 2 out]
        n70 = property on="Particle Concentration from CPC" class="WFChart (strict)"("History Data"=waveform(dbl)[][] []) -> ()  [unwired: 2 in, 2 out]
        n71 = property on="Saving in Progress" class="Slide (strict)"("Caption.Visible"=FALSE) -> ()  [unwired: 2 in, 2 out]
        n72 = property on="Std Error Conc. (%)" class="DigNum (strict)"("NumText.Justify"=w169) -> ()  [unwired: 2 in, 2 out]
        n73 = property on="Running Average Time(sec)" class="DigNum (strict)"("NumText.Justify"=w169) -> ()  [unwired: 2 in, 2 out]
        n74 = property on="Conc. (N/cm^3)" class="DigNum (strict)"("NumText.Justify"=w169) -> ()  [unwired: 2 in, 2 out]
        n75 = property on="Std Conc. error tolerance(%)" class="DigNum (strict)"("NumText.Justify"=w169) -> ()  [unwired: 2 in, 2 out]
        n76 = property on="Mean Conc." class="DigNum (strict)"("NumText.Justify"=w169) -> ()  [unwired: 2 in, 2 out]
        n77 = property on="Std Concentration" class="DigNum (strict)"("NumText.Justify"=w169) -> ()  [unwired: 2 in, 2 out]
        n78 = property on="Std Error Concentration" class="DigNum (strict)"("NumText.Justify"=w169) -> ()  [unwired: 2 in, 2 out]
        n79 = property on="Pressure Graph" class="WFChart (strict)"("History Data"=waveform(dbl)[][] []) -> ()  [unwired: 2 in, 2 out]
        n80 = property on="Temperature Graph" class="WFChart (strict)"("History Data"=waveform(dbl)[][] []) -> ()  [unwired: 2 in, 2 out]
        n81 = call <vilib>:"Add State(s) to Queue__jki_lib_state_machine.vi"("State(s) in (\"\")"=w175) -> ("States Out"=w174:string)  [unwired: 14 in]
      }
      frame "UI: Cursor Set" {
        # "Argument"
        # "Set and Unset Cursor Busy.\n(Usage: \"UI: Cursor Set >> Busy|Idle\")"
        n82 = case shown="\"Idle\", Default" w176 {
          tunnel: w178 -> [w183 w185]
          tunnel: [w182 w184] -> w177
          frame "Idle", Default {
            n83 = call <vilib>:"Unset Busy.vi"("error in (no error)"=w183) -> ("error out"=w182:errorcluster)  [unwired: 10 in]
          }
          frame "Busy" {
            n84 = call <vilib>:"Set Busy.vi"("error in (no error)"=w185) -> ("error out"=w184:errorcluster)  [unwired: 9 in, 1 out]
          }
        }
        n85 = call <vilib>:"Add State(s) to Queue__jki_lib_state_machine.vi"("State(s) in (\"\")"=w181) -> ("States Out"=w180:string)  [unwired: 14 in]
      }
      frame "UI: Front Panel State" {
        # "Argument"
        # "Set Front Panel Open or Closed\n(Usage: \"UI: Front Panel State >> Open|Close\")"
        n86 = Unbundle By Name(w188) -> ("Core.Current VI Reference"=w187:refnum<vi>)
        n87 = case shown="\"Open\", Default" w186 {
          tunnel: w190 -> [w196 w209]
          tunnel: [w198 w210] -> w189
          tunnel: w187 -> [w197 w207]
          frame "Open", Default {
            n88 = property class="VI"(reference=w197, error in=w196) -> (reference out=w194:refnum<vi>, error out=w195:errorcluster, "Front Panel.Open"=w193:bool)
            n89 = case shown="False" w193 {
              tunnel: [w201 w204] -> w198
              tunnel: w195 -> [w200 w204]
              tunnel: w194 -> [w199 _]
              frame False {
                n90 = invoke class="VI" method="FP.Open"(reference=w199, error in=w200, "Activate"=TRUE, "State"=T3."Standard") -> (error out=w201:errorcluster)  [unwired: 1 in, 4 out]
              }
              frame True {
              }
            }
          }
          frame "Close" {
            n91 = property class="VI"(reference=w207, error in=w209) -> (reference out=w206:refnum<vi>, error out=w208:errorcluster, "Front Panel.Open"=w205:bool)
            n92 = case shown="True" w205 {
              tunnel: [w211 w214] -> w210
              tunnel: w208 -> [w211 w213]
              tunnel: w206 -> [_ w212]
              frame False {
              }
              frame True {
                n93 = invoke class="VI" method="FP.Close"(reference=w212, error in=w213) -> (error out=w214:errorcluster)  [unwired: 1 in, 2 out]
              }
            }
          }
        }
        n94 = call <vilib>:"Add State(s) to Queue__jki_lib_state_machine.vi"("State(s) in (\"\")"=w192) -> ("States Out"=w191:string)  [unwired: 14 in]
      }
      frame "---------- Macro ----------" {
        # "Do not put any code in this frame.\n(It is a separator no-op. You can make a copy of this frame to create a new Macro frame)"
        n95 = call <vilib>:"Add State(s) to Queue__jki_lib_state_machine.vi"("State(s) in (\"\")"=w218) -> ("States Out"=w217:string)  [unwired: 14 in]
      }
      frame "Macro: Initialize" {
        w219 = "Data: Initialize\nInitialize Core Data\nUI: Initialize\nUI: Front Panel State >> Open"  # Data: Initialize Initialize Core Data UI: Initialize UI: Front Panel State >> Open
        # "Initialization Macro\n(This is called once, when the VI starts)"
        n96 = call <vilib>:"Add State(s) to Queue__jki_lib_state_machine.vi"("State(s) in Front (\"\")"=w219, "State(s) in (\"\")"=w223) -> ("States Out"=w222:string)  [unwired: 13 in]
      }
      frame "Macro: Exit" {
        # "Exit Macro\n(This is called once, when the VI exits)"
        n97 = Unbundle By Name(w230) -> ("Core.Close Panel on Exit?"=w229:bool)
        n98 = Select(t="UI: Front Panel State >> Close", s=w229, f="") -> (s? t:f=w226:string)
        n99 = call <vilib>:"Add State(s) to Queue__jki_lib_state_machine.vi"("State(s) in (\"\")"=w226, "State(s) at Back (\"\")"="Data: Cleanup\nExit") -> ("States Out"=w224:string)  [unwired: 13 in]
        n100 = call <vilib>:"Add State(s) to Queue__jki_lib_state_machine.vi"("State(s) in Front (\"\")"=w224, "State(s) in (\"\")"=w233) -> ("States Out"=w232:string)  [unwired: 13 in]
      }
      frame "---------- New Category ----------" {
        # "Template Separator\n(You can make a copy of, or modify, this frame)"
        n101 = call <vilib>:"Add State(s) to Queue__jki_lib_state_machine.vi"("State(s) in (\"\")"=w237) -> ("States Out"=w236:string)  [unwired: 14 in]
      }
      frame "Read ConcPressTemp" {
        # "Creates a rotating array for calculation of moving average"
        # "Calculates Mean, std, std error and std error precentages\nand output that results to graph and indicators"
        n102 = call "DAQ Assistant2"() -> ("data"=w268:dynamicdata)  [unwired: 17 in, 2 out]
        n103 = Unbundle(w313) -> (w312:dbl[], "Running Average Time(sec)"=w307:i32, "dup CPC port"=w267:refnum<visa-resource-name>, "CPC model"=w266:string, w296:cluster{dbl[], dbl[], "element":dbl}, w295:cluster{dbl[], dbl[], "element":dbl})  [unwired: 8 out]
        n104 = call "DAQ Assistant"() -> ("data"=w269:dynamicdata)  [unwired: 17 in, 2 out]
        n105 = case shown="\"Gas Measurement\", Default" "Measurment Type" {
          tunnel: w267 -> [_ w321 _]
          tunnel: w266 -> [_ w320 _]
          tunnel: [1.0 ("concentration part/cm3") w319 0.0 ("concentration part/cm3")] -> w265
          frame "Gas Measurement", Default {
          }
          frame "Particles Measurement" {
            n106 = call "CPCReadlior.vi"("model"=w320, "CPC port"=w321) -> ("concentration part/cm3"=w319:dbl)  [unwired: 8 in, 1 out]
          }
          frame "SMPS scan" {
          }
        }
        "Conc. (N/cm^3)" <- w265
        "CPCconc" <- w265
        n107 = call "Convert from Dynamic Data2"("Dynamic Data Type"=w268) -> ("Scalar"=w241:dbl)  [unwired: 3 in]
        "P (Hectopascal)" <- w241
        n108 = Unbundle(w296) -> (w293:dbl[], w286:dbl[])  [unwired: 1 out]
        n109 = Unbundle(w295) -> (w291:dbl[], w284:dbl[])  [unwired: 1 out]
        n110 = Rotate 1D Array(1:w312, 2:1 ("n")) -> (0:w310:dbl[])
        n111 = Rotate 1D Array(1:w293, 2:1 ("n")) -> (0:w290:dbl[])
        n112 = Rotate 1D Array(1:w291, 2:1 ("n")) -> (0:w288:dbl[])
        n113 = call "Convert from Dynamic Data"("Dynamic Data Type"=w269) -> ("Scalar"=w240:dbl)  [unwired: 3 in]
        "Temp (C)" <- w240
        n114 = Replace Array Subset(array=w310, new element=w265, index=0.0 ("new element/subarray")) -> (w302:dbl[])
        "output array" <- w302
        n115 = Less?(x=w307, y=0) -> (x < y?=w270:bool)
        n116 = case shown="False" w270 {
          tunnel: w265 -> [w347 w350]
          tunnel: w302 -> [_ w356]
          tunnel: [w348 w357] -> w301
          tunnel: [w348 w349] -> w299
          tunnel: [w348 w353] -> w305
          tunnel: [w348 w351] -> w300
          tunnel: [w347 w350] -> w244
          tunnel: [w347 w349] -> w243
          frame False {
            w348 = 0 ("y")
          }
          frame True {
            n117 = Array Size(array=w356) -> (size(s)=w355:i32)
            n118 = Square Root(x=w355) -> (sqrt(x)=w354:dbl)
            n119 = call <vilib>:"Std Deviation and Variance.vi"("X"=w356) -> ("mean"=w349:dbl, "standard deviation"=w353:dbl)  [unwired: 1 in, 1 out]
            n120 = Divide(x=w353, y=w354) -> (x/y=w351:dbl)
            n121 = Divide(x=w351, y=w349) -> (x/y=w352:dbl)
            n122 = Multiply(x=w352, y=100.0) -> (x*y=w357:dbl)
          }
        }
        "Std Error Conc. (%)" <- w301
        "Mean Conc." <- w299
        "Std Concentration" <- w305
        "Std Error Concentration" <- w300
        n123 = Replace Array Subset(array=w290, new element=w241, index=0) -> (w282:dbl[])
        n124 = Replace Array Subset(array=w288, new element=w240, index=0) -> (w281:dbl[])
        n125 = case shown="True" w270 {
          tunnel: w241 -> [w335 w338]
          tunnel: w282 -> [_ w344]
          tunnel: [w336 w345] -> w277
          tunnel: [w336 w337] -> w239
          tunnel: [w336 w341] -> _
          tunnel: [w336 w339] -> _
          tunnel: [w335 w338] -> w257
          tunnel: [w335 w337] -> w255
          frame False {
            w336 = 0 ("y")
          }
          frame True {
            n126 = Array Size(array=w344) -> (size(s)=w343:i32)
            n127 = call <vilib>:"Std Deviation and Variance.vi"("X"=w344) -> ("mean"=w337:dbl, "standard deviation"=w341:dbl)  [unwired: 1 in, 1 out]
            n128 = Square Root(x=w343) -> (sqrt(x)=w342:dbl)
            n129 = Divide(x=w341, y=w342) -> (x/y=w339:dbl)
            n130 = Divide(x=w339, y=w337) -> (x/y=w340:dbl)
            n131 = Multiply(x=w340, y=100.0) -> (x*y=w345:dbl)
          }
        }
        "Mean P" <- w239
        "Std Error P (%)" <- w277
        "CavityPressure" <- w239
        n132 = case shown="True" w270 {
          tunnel: w240 -> [w323 w326]
          tunnel: w281 -> [_ w332]
          tunnel: [w324 w333] -> w272
          tunnel: [w324 w325] -> w238
          tunnel: [w324 w329] -> _
          tunnel: [w324 w327] -> _
          tunnel: [w323 w326] -> w263
          tunnel: [w323 w325] -> w260
          frame False {
            w324 = 0 ("y")
          }
          frame True {
            n133 = Array Size(array=w332) -> (size(s)=w331:i32)
            n134 = Square Root(x=w331) -> (sqrt(x)=w330:dbl)
            n135 = call <vilib>:"Std Deviation and Variance.vi"("X"=w332) -> ("mean"=w325:dbl, "standard deviation"=w329:dbl)  [unwired: 1 in, 1 out]
            n136 = Divide(x=w329, y=w330) -> (x/y=w327:dbl)
            n137 = Divide(x=w327, y=w325) -> (x/y=w328:dbl)
            n138 = Multiply(x=w328, y=100.0) -> (x*y=w333:dbl)
          }
        }
        "Std Error T (%)" <- w272
        "Mean Temp" <- w238
        "CavityTemperature" <- w238
        n139 = Decrement(x=w307) -> (x-1=w308:i32)
        n140 = Bundle(w282, w286, "Scalar"=w241) -> (w285:cluster{dbl[], dbl[], "Scalar":dbl})  [unwired: 1 in]
        n141 = Bundle(w281, w284, "Scalar"=w240) -> (w283:cluster{dbl[], dbl[], "Scalar":dbl})  [unwired: 1 in]
        n142 = Bundle(cluster=w313, w302, "Running Average Time(sec)"=w308, "element"=w265, w285, w283) -> (w314:T4)  [unwired: 9 in]
        n143 = Get Date/Time In Seconds() -> (seconds since 1Jan1904=w250:timestamp)
        n144 = Build Array(w263) -> (w262:dbl[])
        n145 = Build Array(w260) -> (w259:dbl[])
        n146 = Greater?(x="Std Press. error tolerance(%)", y=w277) -> (0:w280:bool)
        n147 = Greater?(x="Std Temp error tolerance(%)", y=w272) -> (0:w275:bool)
        n148 = Bundle By Name("Y"=w259, "t0"=w250) -> (w258:waveform(dbl))  [unwired: 1 in]
        n149 = Bundle By Name("Y"=w262, "t0"=w250) -> (w264:waveform(dbl))  [unwired: 1 in]
        n150 = And(x=w280, y=w270) -> (x .and. y?=w279:bool)
        n151 = And(x=w275, y=w270) -> (x .and. y?=w274:bool)
        n152 = Build Array(w264, w258) -> (→"Temperature Graph":waveform(dbl)[])
        n153 = Greater?(x="Std Conc. error tolerance(%)", y=w301) -> (0:w303:bool)
        n154 = Not(x=w279) -> (.not. x?=w276:bool)
        n155 = Not(x=w274) -> (.not. x?=w271:bool)
        n156 = property on="Mean P" class="DigNum (strict)"("Blinking"=w276) -> ()  [unwired: 2 in, 2 out]
        n157 = property on="Mean Temp" class="DigNum (strict)"("Blinking"=w271) -> ()  [unwired: 2 in, 2 out]
        n158 = And(x=w303, y=w270) -> (x .and. y?=w298:bool)
        n159 = Build Array(w255) -> (w254:dbl[])
        n160 = Build Array(w257) -> (w256:dbl[])
        n161 = Build Array(w244) -> (w249:dbl[])
        n162 = Build Array(w243) -> (w248:dbl[])
        n163 = Bundle By Name("Y"=w249, "t0"=w250) -> (w247:waveform(dbl))  [unwired: 1 in]
        n164 = Bundle By Name("Y"=w248, "t0"=w250) -> (w246:waveform(dbl))  [unwired: 1 in]
        n165 = Bundle By Name("Y"=w256, "t0"=w250) -> (w253:waveform(dbl))  [unwired: 1 in]
        n166 = Bundle By Name("Y"=w254, "t0"=w250) -> (w252:waveform(dbl))  [unwired: 1 in]
        n167 = Not(x=w298) -> (.not. x?=w297:bool)
        n168 = Build Array(w247, w246) -> (→"Particle Concentration from CPC":waveform(dbl)[])
        n169 = Build Array(w253, w252) -> (→"Pressure Graph":waveform(dbl)[])
        n170 = property on="Mean Conc." class="DigNum (strict)"("Blinking"=w297) -> ()  [unwired: 2 in, 2 out]
        n171 = call <vilib>:"Add State(s) to Queue__jki_lib_state_machine.vi"("State(s) in (\"\")"=w317) -> ("States Out"=w316:string)  [unwired: 14 in]
      }
      frame "New Category: 2" {
        # "Your code here.\n(You can make a copy of, or modify, this frame)"
        n172 = call <vilib>:"Add State(s) to Queue__jki_lib_state_machine.vi"("State(s) in (\"\")"=w362) -> ("States Out"=w361:string)  [unwired: 14 in]
      }
      frame "Take Measurement" {
        # "Incase andor script is aborted\ninitiate a timeout of 3 min in recording the data and reinitialize to zero"
        # "Your code here.\n(You can make a copy of, or modify, this frame)"
        n173 = Unbundle(w386) -> (w387:dbl[], "element"=w389:dbl, w374:cluster{dbl[], dbl[], "element":dbl}, w373:cluster{dbl[], dbl[], "element":dbl})  [unwired: 10 out]
        n174 = property on="Saving in Progress" class="Slide (strict)"("Caption.Visible"=TRUE) -> ()  [unwired: 2 in, 2 out]
        n175 = Unbundle(w374) -> (w368:dbl[], w372:dbl[], "element"=w369:dbl)
        n176 = Unbundle(w373) -> (w365:dbl[], w371:dbl[], "element"=w364:dbl)
        n177 = Insert Into Array(array=w387, index=0, new element=w389) -> (w384:dbl[])
        "output array 2" <- w384
        n178 = Insert Into Array(array=w372, index=0, new element=w369) -> (w370:dbl[])
        n179 = Insert Into Array(array=w371, index=0, new element=w364) -> (w366:dbl[])
        n180 = Array Size(array=w384) -> (size(s)=w380:i32)
        n181 = Bundle(w368, w370, "element"=w369) -> (w367:cluster{dbl[], dbl[], "element":dbl})  [unwired: 1 in]
        n182 = Bundle(w365, w366, "element"=w364) -> (w363:cluster{dbl[], dbl[], "element":dbl})  [unwired: 1 in]
        n183 = Quotient & Remainder(x=w380, y=10) -> (x-y*floor(x/y)=→"Saving in Progress":i32)  [unwired: 1 out]
        n184 = Greater?(x=w380, y=300) -> (0:w378:bool)
        n185 = Bundle(cluster=w386, w384, "dimension size"=w380, w367, w363) -> (w385:T4)  [unwired: 10 in]
        n186 = case shown="True" w378 {
          tunnel: ["" ("State(s) in Front (\"\")") "Write to file" ("State(s) in Front (\"\")")] -> w377
          frame False {
          }
          frame True {
          }
        }
        n187 = call <vilib>:"Add State(s) to Queue__jki_lib_state_machine.vi"("State(s) in Front (\"\")"=w377, "State(s) in (\"\")"=w392) -> ("States Out"=w391:string)  [unwired: 13 in]
      }
      frame "Write to file" {
        # "Initialize mean after it is written to file"
        n188 = Unbundle(w441) -> (w449:dbl[], "input file"=w432:path, "input file"=w433:path, "input file"=w419:path, "input file"=w418:path, w429:cluster{dbl[], dbl[], "element":dbl}, w428:cluster{dbl[], dbl[], "element":dbl})  [unwired: 7 out]
        n189 = property on="Saving in Progress" class="Slide (strict)"("Caption.Visible"=FALSE) -> ()  [unwired: 2 in, 2 out]
        n190 = property on="Saving in Progress" class="Slide (strict)"("Value"=0 ("Saving in Progress")) -> ()  [unwired: 2 in, 2 out]
        n191 = Array Size(array=w449) -> (size(s)=w446:i32)
        "Number Samples of Conc." <- w446
        n192 = Delete(path (use dialog)=w432, error in=w430) -> (deleted path=w431:path, error out=w416:errorcluster)  [unwired: 3 in, 1 out]
        n193 = Delete(path (use dialog)=w419, error in=w416) -> (deleted path=w411:path, error out=w417:errorcluster)  [unwired: 3 in, 1 out]
        n194 = Delete(path (use dialog)=w418, error in=w417) -> (deleted path=w407:path, error out=w415:errorcluster)  [unwired: 3 in, 1 out]
        n195 = call <vilib>:"Std Deviation and Variance.vi"("X"=w449) -> ("mean"=w444:dbl, "standard deviation"=w448:dbl)  [unwired: 1 in, 1 out]
        "Mean conc. to file (N/cm^3)" <- w444
        n196 = Unbundle(w429) -> (w406:dbl[], w427:dbl[], "element"=w405:dbl)
        n197 = Unbundle(w428) -> (w404:dbl[], w422:dbl[], "element"=w403:dbl)
        n198 = Format Into String(format string="%d %d", initial string=w433, 0.0 ("input 1"), 0.0 ("input 2")) -> ()  [unwired: 1 in, 2 out]
        n199 = Array Size(array=w427) -> (size(s)=w420:i32)
        "Number Samples of Press." <- w420
        n200 = call <vilib>:"Std Deviation and Variance.vi"("X"=w427) -> ("mean"=w413:dbl, "standard deviation"=w425:dbl)  [unwired: 1 in, 1 out]
        "Mean Press. to file (hpas)" <- w413
        n201 = Square Root(x=w446) -> (sqrt(x)=w450:dbl)
        n202 = Array Size(array=w422) -> (size(s)=w421:i32)
        "Number Samples of Temp" <- w421
        n203 = call <vilib>:"Std Deviation and Variance.vi"("X"=w422) -> ("mean"=w409:dbl, "standard deviation"=w423:dbl)  [unwired: 1 in, 1 out]
        "Mean Temp to file (deg)" <- w409
        n204 = Square Root(x=w420) -> (sqrt(x)=w426:dbl)
        n205 = Square Root(x=w421) -> (sqrt(x)=w424:dbl)
        n206 = Divide(x=w448, y=w450) -> (x/y=w445:dbl)
        "Std error to file (N/cm^3)" <- w445
        n207 = Divide(x=w425, y=w426) -> (x/y=w412:dbl)
        "Std error Press. to file (hpas)" <- w412
        n208 = Divide(x=w423, y=w424) -> (x/y=w408:dbl)
        "Std error Temp to file (deg)" <- w408
        n209 = Format Into String(format string="%f, %f,", initial string=w431, w444, w445) -> ()  [unwired: 1 in, 2 out]
        n210 = Format Into String(format string="%f, %f,", initial string=w411, w413, w412) -> ()  [unwired: 1 in, 2 out]
        n211 = Format Into String(format string="%f, %f,", initial string=w407, w409, w408) -> ()  [unwired: 1 in, 2 out]
        n212 = Initialize Array(0.0 ("element"), 0 ("dimension size")) -> (w400:dbl[])
        n213 = Initialize Array(0.0 ("element"), 0 ("dimension size")) -> (w397:dbl[])
        n214 = Bundle(w404, w400, "element"=w403) -> (w395:cluster{dbl[], dbl[], "element":dbl})  [unwired: 1 in]
        n215 = Bundle(w406, w397, "element"=w405) -> (w396:cluster{dbl[], dbl[], "element":dbl})  [unwired: 1 in]
        n216 = Initialize Array(0.0 ("element"), 0 ("dimension size")) -> (w439:dbl[])
        n217 = Bundle(cluster=w441, w439, w396, w395) -> (w440:T4)  [unwired: 11 in]
        n218 = call <vilib>:"Add State(s) to Queue__jki_lib_state_machine.vi"("State(s) in (\"\")"=w452) -> ("States Out"=w451:string)  [unwired: 14 in]
      }
    }
  }
